vi "getColor.vi"(8 "error in (no error)":errorcluster, 10 "Color":string, 11 "AbstractFactory in":refnum<class "AbstractFactory.lvclass">) -> (0 "error out":errorcluster, 2 "afColor.lvclass":refnum<class "afColor.lvclass">, 3 "AbstractFactory out":refnum<class "AbstractFactory.lvclass">)   [LabVIEW 2017, in "AbstractFactory.lvclass"]
uses:
  AbstractFactory.lvclass
  afColor Class/afColor.lvclass
  AbstractFactory.lvclass/AbstractFactory.ctl
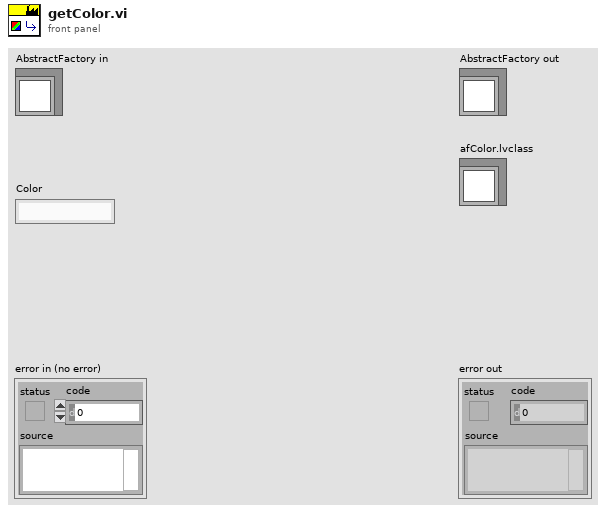
[diagram p1: front panel]
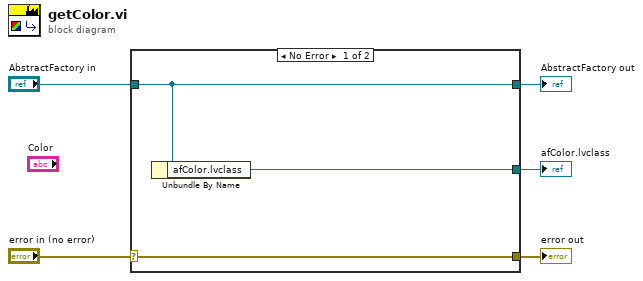
[diagram p0: block diagram]
diagram:
  n1 = case shown="No Error" "error in (no error)" {
    selector: "error in (no error)" -> [w8 w9]
    tunnel: [w8 w9] -> w4
    tunnel: [w7 w10] -> w2
    tunnel: "AbstractFactory in" -> [w7 w10]
    tunnel: [w6 _] -> w1
    frame No Error {
      n2 = Unbundle By Name(w7) -> ("afColor.lvclass"=w6:refnum<class "afColor.lvclass">)
    }
    frame Error {
    }
  }
  "error out" <- w4
  "AbstractFactory out" <- w2
  "afColor.lvclass" <- w1
